vi "test-quintic-spline-01.vi"() -> (3 "Test Passed":bool)   [LabVIEW 2019]
uses:
  <vilib>/Rock Robotics/WPI/ThirdParty/JAS_Junk/TrajLib/TRANSLATION2D.ctl
  <vilib>/Rock Robotics/WPI/ThirdParty/JAS_Junk/TrajLib/Trajectory_Library.lvlib
  <vilib>/Rock Robotics/WPI/ThirdParty/JAS_Junk/TrajLib/ROTATION2D.ctl
  <vilib>/Rock Robotics/WPI/ThirdParty/JAS_Junk/TrajLib/POSE2D.ctl
  <vilib>/Rock Robotics/WPI/ThirdParty/JAS_Junk/TrajLib/POSEwCURVATURE.ctl
panel:
  out "XY Graph":cluster{dbl[], dbl[]}(graph)
  out "Numb\nWaypoints":i32
  out "All Interior \nwayPoints\nFound (True)":bool
  out "end rot = 0":dbl
  out "end y = 0":dbl
  out "end x = 0":dbl
  out "start rot = 0":dbl
  out "start y = 0":dbl
  out "start x = 0":dbl
  out "max dtheta < 0.0872":dbl
  out "max dy < 0.00127":dbl
  out "max dx  < 0.127":dbl
  out "Overall Error":errorcluster
  out "Elements":i32
  out "Create Spline Error":errorcluster
  out "SplinePoses\nWCurve":T1[](array[typedef]) {"POSE"."ROTATION"."SIN" format="%13.4f"; "POSE"."ROTATION"."COS" format="%13.4f"; "POSE"."ROTATION"."VALUE" format="%13.4f"; "POSE"."TRANSLATION"."Y" format="%14.3f"; "POSE"."TRANSLATION"."X" format="%14.3f"}
  out "Elapsed Time":dbl
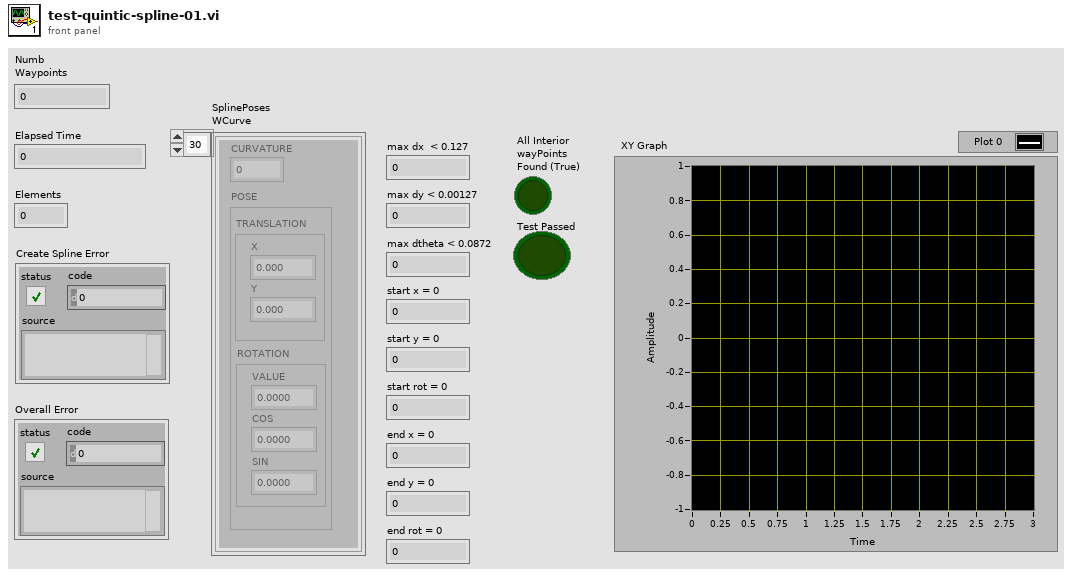
[diagram p1: front panel]
types:
  T1 = typedef "Trajectory_Library.lvlib/POSEwCURVATURE.ctl" = cluster{"CURVATURE":dbl, "POSE":T2}
  T2 = typedef "Trajectory_Library.lvlib/POSE2D.ctl" = cluster{"TRANSLATION":T3, "ROTATION":T4}
  T3 = typedef "Trajectory_Library.lvlib/TRANSLATION2D.ctl" = cluster{"X":dbl, "Y":dbl}
  T4 = typedef "Trajectory_Library.lvlib/ROTATION2D.ctl" = cluster{"VALUE":dbl, "COS":dbl, "SIN":dbl}
  T5 = typedef "Trajectory_Library.lvlib/SPLINE_CTRL_VECTOR.ctl" = cluster{"Xs":dbl[], "Ys":dbl[]}
  T6 = typedef "Trajectory_Library.lvlib/SPLINE.ctl" = cluster{"Degree":i32, "Coefficients":T7}
  T7 = typedef "NI_Matrix.lvlib/RealMatrix.ctl" = dbl[][]
  T8 = typedef "Trajectory_Library.lvlib/TWIST2D.ctl" = cluster{"dX":dbl, "dY":dbl, "dTHETA":dbl}
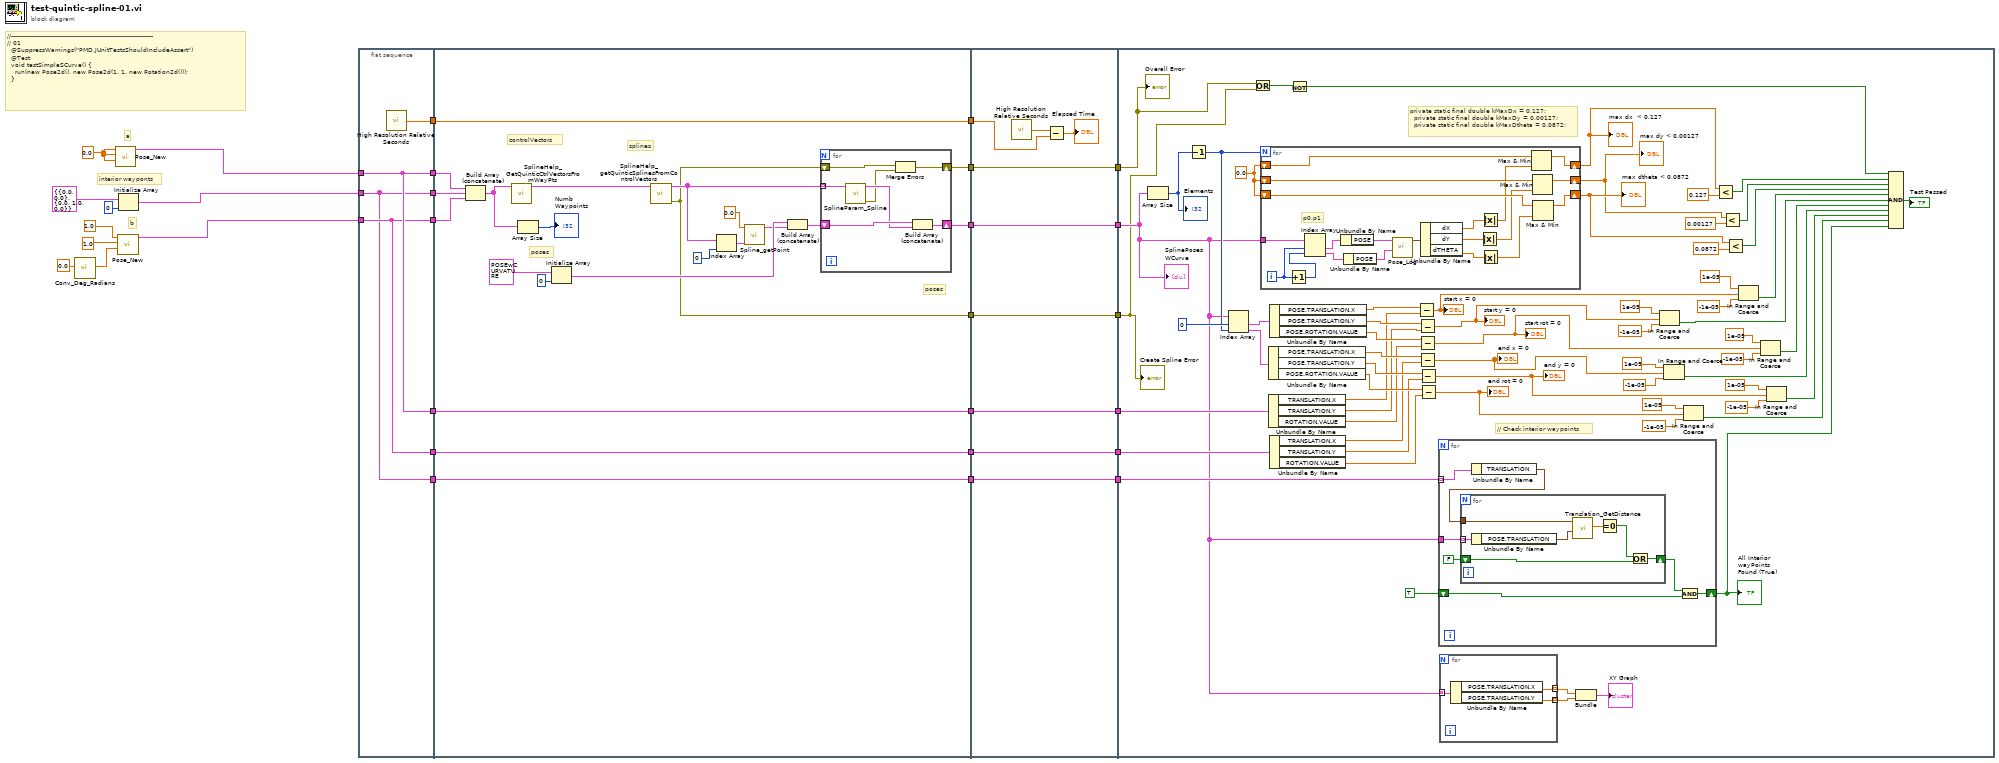
[diagram p0: block diagram]
diagram:
  w10 = 0.0 ("X")
  # "interior wayponts"
  # "b"
  # "a"
  # "//-----------------------------------------------------------------------\n// 01\n  @SuppressWarnings(\"PMD.JUnitTestsShouldIncludeAssert\")\n  @Test\n  void testSimpleSCurve() {\n    run(new Pose2d(), new Pose2d(1, 1, new Rotation2d()));\n  }"
  n1 = call <vilib>:"Conv_Deg_Radians.vi"("Degress"=0.0) -> ("Radians"=w5:dbl)  [unwired: 10 in]
  n2 = call <vilib>:"Pose_New.vi"("Heading"=w10, "Y"=w10, "X"=w10) -> ("out POSe"=w3:T2)  [unwired: 8 in]
  n3 = call <vilib>:"Pose_New.vi"("Heading"=w5, "Y"=1.0, "X"=1.0) -> ("out POSe"=w1:T2)  [unwired: 8 in]
  n4 = Initialize Array(T2 {"TRANSLATION"={"X"=0.0, "Y"=0.0}, "ROTATION"={"VALUE"=0.0, "COS"=1.0, "SIN"=0.0}} ("POSE"), 0 ("dimension size")) -> (w2:T2[])
  n5 = flat-sequence {
    tunnel: w3 -> [w33]
    tunnel: [w33] -> w30
    tunnel: w1 -> [w32]
    tunnel: [w32] -> w29
    tunnel: [w34] -> w28
    tunnel: [w33] -> w20
    tunnel: [w32] -> w17
    tunnel: [w31] -> w12
    tunnel: w2 -> [w31]
    tunnel: [w31] -> w11
    tunnel: w30 -> [w40]
    tunnel: w29 -> [w38]
    tunnel: [w56] -> w27
    tunnel: w28 -> [w56]
    tunnel: [w46] -> w26
    tunnel: [w45] -> w24
    tunnel: [w44] -> w22
    tunnel: w20 -> [w43]
    tunnel: [w43] -> w19
    tunnel: w17 -> [w42]
    tunnel: [w42] -> w16
    tunnel: [w41] -> w13
    tunnel: w12 -> [w41]
    tunnel: w11 -> [w35]
    tunnel: w27 -> [w72]
    tunnel: w26 -> [w71]
    tunnel: [w71] -> w25
    tunnel: w24 -> [w70]
    tunnel: [w70] -> w23
    tunnel: w22 -> [w69]
    tunnel: [w69] -> w21
    tunnel: w19 -> [w66]
    tunnel: [w66] -> w18
    tunnel: w16 -> [w65]
    tunnel: [w65] -> w15
    tunnel: [w64] -> w14
    tunnel: w13 -> [w64]
    tunnel: w25 -> [w113]
    tunnel: w23 -> [w100]
    tunnel: w21 -> [w99]
    tunnel: w18 -> [w135]
    tunnel: w15 -> [w134]
    tunnel: w14 -> [w117]
    frame #0 {
      n6 = call <vilib>:"High Resolution Relative Seconds.vi"() -> ("relative seconds"=w34:dbl)
    }
    frame #1 {
      # "poses"
      # "poses"
      # "splines"
      # "controlVectors"
      n7 = Build Array (concatenate)(w40, w35, w38) -> (w37:T2[])
      n8 = call <vilib>:"SplineHelp_GetQuinticCtrlVectorsFromWayPts.vi"("WayPoints"=w37) -> ("SplineControlVectors"=w39:T5[])  [unwired: 10 in]
      n9 = Array Size(array=w37) -> (size(s)=→"Numb\nWaypoints":i32)
      n10 = Initialize Array(T1 {"CURVATURE"=0.0, "POSE"={"TRANSLATION"={"X"=0.0, "Y"=0.0}, "ROTATION"={"VALUE"=0.0, "COS"=1.0, "SIN"=0.0}}} ("POSEwCURVATURE"), 0 ("dimension size")) -> (w50:T1[])
      n11 = call <vilib>:"SplineHelp_getQuinticSplinesFromControlVectors.vi"("ControlVectors"=w39) -> ("error out"=w45:errorcluster, "splines"=w47:T6[])  [unwired: 9 in]
      n12 = Index Array(array=w47, index=0) -> (element=w52:T6)
      n13 = call <vilib>:"Spline_getPoint.vi"("inputSPLINE"=w52, "Time"=0.0) -> ("POSEwCURVATURE"=w49:T1)  [unwired: 9 in]
      n14 = Build Array (concatenate)(w50, w49) -> (w48:T1[])
      n15 = for {
        shift-right: [w60] -> w46
        shift-left: w48 -> [w62]
        tunnel: w47 -> [w63] mode=indexing
        shift-right: [w58] -> w44
        shift-left: w45 -> [w59]
        n16 = call <vilib>:"SplineParam_Spline.vi"("inputSPLINE"=w63) -> ("error out"=w57:errorcluster, "outputPOSEwCURVATURE"=w61:T1[])  [unwired: 9 in]
        n17 = Merge Errors(w59, w57) -> (w58:errorcluster)
        n18 = Build Array (concatenate)(w62, w61) -> (w60:T1[])
      }
    }
    frame #2 {
      n19 = call <vilib>:"High Resolution Relative Seconds.vi"() -> ("relative seconds"=w67:dbl)
      n20 = Subtract(x=w67, y=w72) -> (x-y=→"Elapsed Time":dbl)
    }
    frame #3 {
      w136 = 0.0
      # "// Check interior waypoints"
      # "private static final double kMaxDx = 0.127;\n  private static final double kMaxDy = 0.00127;\n  private static final double kMaxDtheta = 0.0872;"
      n21 = Array Size(array=w113) -> (size(s)=w137:i32)
      "Elements" <- w137
      n22 = Decrement(x=w137) -> (x-1=w132:i32)
      n23 = Index Array(array=w113, index #1=0 ("index"), index #2=w132) -> (element #1=w131:T1, element #2=w130:T1)
      n24 = Or(x=w99, y=w100) -> (x .or. y?=w101:bool)
      n25 = for {
        N: w132 -> [_]
        tunnel: w113 -> [w172]
        shift-right: [w163] -> w105
        shift-left: w136 -> [w160]
        shift-right: [w161] -> w107
        shift-left: w136 -> [w158]
        shift-right: [w162] -> w106
        shift-left: w136 -> [w159]
        i -> [w174]
        # "p0,p1"
        n26 = Increment(x=w174) -> (x+1=w173:i32)
        n27 = Index Array(array=w172, index #1=w174, index #2=w173) -> (element #1=w171:T1, element #2=w170:T1)
        n28 = Unbundle By Name(w171) -> ("POSE"=w169:T2)
        n29 = Unbundle By Name(w170) -> ("POSE"=w168:T2)
        n30 = call <vilib>:"Pose_Log.vi"("end POSE"=w168, "in POSE"=w169) -> ("out TWIST"=w167:T8)  [unwired: 9 in]
        n31 = Unbundle By Name(w167) -> ("dX"=w164:dbl, "dY"=w165:dbl, "dTHETA"=w166:dbl)
        n32 = Absolute Value(x=w165) -> (abs(x)=w156:dbl)
        n33 = Absolute Value(x=w164) -> (abs(x)=w157:dbl)
        n34 = Absolute Value(x=w166) -> (abs(x)=w155:dbl)
        n35 = Max & Min(x=w160, y=w157) -> (max(x,y)=w163:dbl)  [unwired: 1 out]
        n36 = Max & Min(x=w159, y=w156) -> (max(x,y)=w162:dbl)  [unwired: 1 out]
        n37 = Max & Min(x=w158, y=w155) -> (max(x,y)=w161:dbl)  [unwired: 1 out]
      }
      "max dx  < 0.127" <- w105
      "max dy < 0.00127" <- w106
      "max dtheta < 0.0872" <- w107
      n38 = Unbundle By Name(w130) -> ("POSE.TRANSLATION.X"=w126:dbl, "POSE.TRANSLATION.Y"=w125:dbl, "POSE.ROTATION.VALUE"=w124:dbl)
      n39 = Unbundle By Name(w135) -> ("TRANSLATION.X"=w123:dbl, "TRANSLATION.Y"=w122:dbl, "ROTATION.VALUE"=w121:dbl)
      n40 = Unbundle By Name(w131) -> ("POSE.TRANSLATION.X"=w129:dbl, "POSE.TRANSLATION.Y"=w128:dbl, "POSE.ROTATION.VALUE"=w127:dbl)
      n41 = Unbundle By Name(w134) -> ("TRANSLATION.X"=w120:dbl, "TRANSLATION.Y"=w119:dbl, "ROTATION.VALUE"=w118:dbl)
      n42 = Not(x=w101) -> (.not. x?=w98:bool)
      n43 = Subtract(x=w129, y=w123) -> (x-y=w94:dbl)
      "start x = 0" <- w94
      n44 = Subtract(x=w128, y=w122) -> (x-y=w73:dbl)
      "start y = 0" <- w73
      n45 = Subtract(x=w127, y=w121) -> (x-y=w77:dbl)
      "start rot = 0" <- w77
      n46 = Subtract(x=w126, y=w120) -> (x-y=w78:dbl)
      "end x = 0" <- w78
      n47 = Subtract(x=w125, y=w119) -> (x-y=w85:dbl)
      "end y = 0" <- w85
      n48 = Subtract(x=w124, y=w118) -> (x-y=w89:dbl)
      "end rot = 0" <- w89
      n49 = for {
        tunnel: w117 -> [w142] mode=indexing
        tunnel: w113 -> [w147]
        shift-right: [w146] -> w97
        shift-left: TRUE -> [w145]
        n50 = Unbundle By Name(w142) -> ("TRANSLATION"=w141:T3)
        n51 = for {
          tunnel: w147 -> [w151] mode=indexing
          shift-right: [w154] -> w143
          shift-left: FALSE -> [w153]
          tunnel: w141 -> [w152]
          n52 = Unbundle By Name(w151) -> ("POSE.TRANSLATION"=w150:T3)
          n53 = call <vilib>:"Translation_GetDistance.vi"("other Translation"=w150, "In Translation"=w152) -> ("Distance"=w149:dbl)  [unwired: 9 in]
          n54 = Equal To 0?(x=w149) -> (x = 0?=w148:bool)
          n55 = Or(x=w148, y=w153) -> (x .or. y?=w154:bool)
        }
        n56 = And(x=w143, y=w145) -> (x .and. y?=w146:bool)
      }
      "All Interior \nwayPoints\nFound (True)" <- w97
      n57 = for {
        tunnel: [w140] -> w115 mode=indexing
        tunnel: [w139] -> w114 mode=indexing
        tunnel: w113 -> [w138] mode=indexing
        n58 = Unbundle By Name(w138) -> ("POSE.TRANSLATION.X"=w140:dbl, "POSE.TRANSLATION.Y"=w139:dbl)
      }
      n59 = Bundle(w115, w114) -> (→"XY Graph":cluster{dbl[], dbl[]})  [unwired: 1 in]
      n60 = In Range and Coerce(upper limit=1e-05, x=w73, lower limit=-1e-05) -> (In Range?=w74:bool)  [unwired: 1 out]
      n61 = In Range and Coerce(upper limit=1e-05, x=w78, lower limit=-1e-05) -> (In Range?=w80:bool)  [unwired: 1 out]
      n62 = In Range and Coerce(upper limit=1e-05, x=w89, lower limit=-1e-05) -> (In Range?=w90:bool)  [unwired: 1 out]
      n63 = Less?(x=w105, y=0.127) -> (x < y?=w104:bool)
      n64 = Less?(x=w106, y=0.00127) -> (x < y?=w103:bool)
      n65 = Less?(x=w107, y=0.0872) -> (x < y?=w102:bool)
      n66 = In Range and Coerce(upper limit=1e-05, x=w94, lower limit=-1e-05) -> (In Range?=w93:bool)  [unwired: 1 out]
      n67 = In Range and Coerce(upper limit=1e-05, x=w77, lower limit=-1e-05) -> (In Range?=w79:bool)  [unwired: 1 out]
      n68 = In Range and Coerce(upper limit=1e-05, x=w85, lower limit=-1e-05) -> (In Range?=w86:bool)  [unwired: 1 out]
      n69 = Compound Arithmetic op=AND(w98, w104, w103, w102, w93, w74, w79, w80, w86, w90, w97) -> (→"Test Passed":bool)
      "SplinePoses\nWCurve" <- w113
      "Create Spline Error" <- w100
      "Overall Error" <- w99
    }
  }
